vi "Commands.vi"() -> ()   [LabVIEW 2014]
panel:
  in  "Enum":T1(ring)
  in  "Send Command":bool
  out "CheckSum Success":bool
  out "Open Comport Error":bool
  out "ACK Receive Error":bool
  out "Command Sent Error":bool
  out "Response Receive Error":bool
  out "Close Comport Error":bool
  out "ASCII String":string
  out "HEX String":string
  in  "VISA resource name":refnum<visa-resource-name>="COM1"
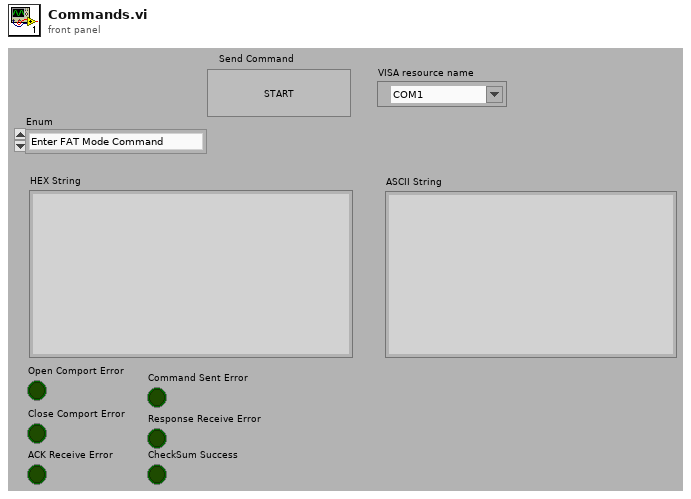
[diagram p1: front panel]
types:
  T1 = enum16{"Enter FAT Mode Command", "Enter Bootstrap Mode Command"}
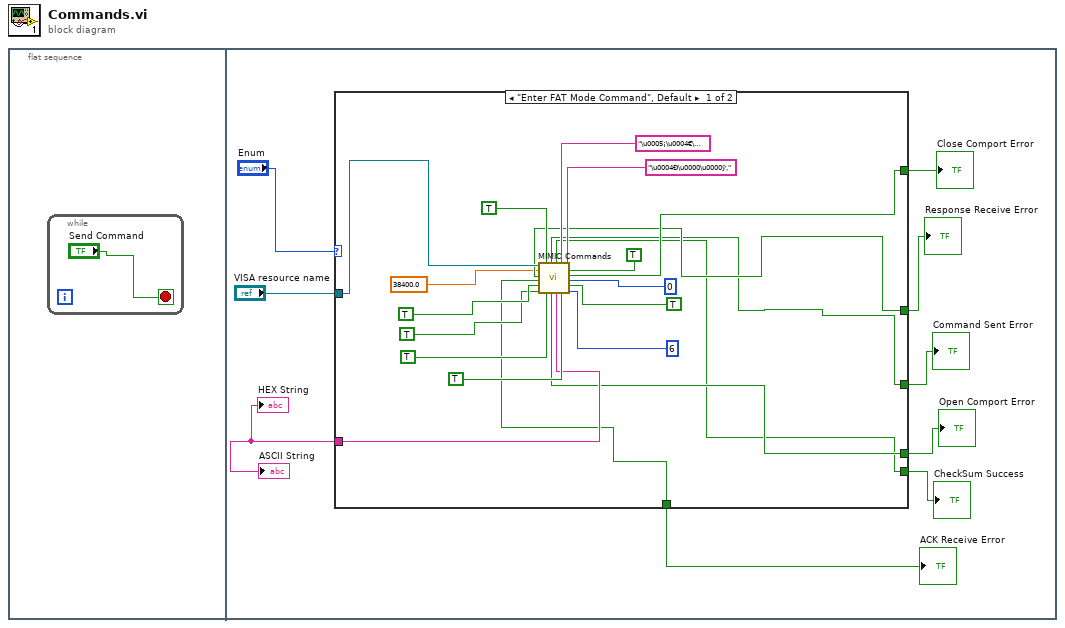
[diagram p0: block diagram]
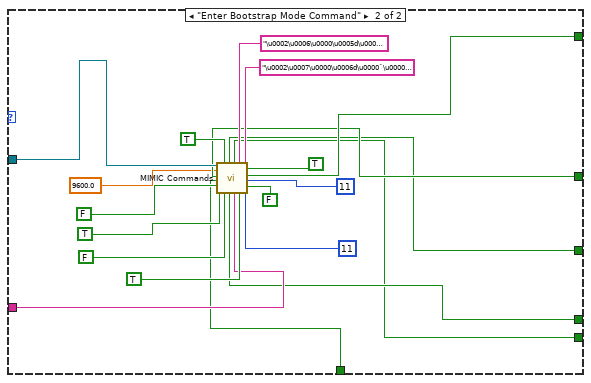
[diagram p2: hidden frame]
diagram:
  n1 = flat-sequence {
    frame #0 {
      n2 = while {
        stop <- "Send Command" stop-if-true
      }
    }
    frame #1 {
      n3 = case shown="\"Enter FAT Mode Command\", Default" "Enum" {
        tunnel: "VISA resource name" -> [w19 w39]
        tunnel: [w18 w38] -> w9
        tunnel: [w17 w37] -> w8
        tunnel: [w16 w36] -> w7
        tunnel: [w15 w35] -> w6
        tunnel: [w14 w34] -> w5
        tunnel: [w13 w33] -> w4
        tunnel: [w12 w32] -> w3
        frame "Enter FAT Mode Command", Default {
          n4 = call "MIMIC Commands.vi"("VISA resource name"=w19, "Baud Rate"=38400.0, "Verify CheckSum"=TRUE, "Read COM Port"=TRUE, "Write to COM Port"=TRUE, "Add CheckSum"=TRUE, "String To Write"="\u0005¡\u0004€\u0010", "Send Command"=TRUE, "ACK HEX String"="\u0004Ð\u0000\u0000ÿ,", "ACK"=TRUE, "Response: bytes to\n read"=u32 0 ("Response: bytes to\n read"), "Response"=TRUE, "ACK: bytes to read"=u32 6) -> ("Response RECEIVE ERROR"=w16:bool, "ACK RECEIVE Error"=w12:bool, "Command SENT Error"=w15:bool, "Open Comport Error"=w14:bool, "CheckSum SUCCESS"=w13:bool, "Response HEX String"=w18:string, "Close Comport Error"=w17:bool)
        }
        frame "Enter Bootstrap Mode Command" {
          n5 = call "MIMIC Commands.vi"("VISA resource name"=w39, "Baud Rate"=9600.0, "Verify CheckSum"=FALSE, "Read COM Port"=TRUE, "Write to COM Port"=TRUE, "Add CheckSum"=FALSE, "String To Write"="\u0002\u0006\u0000\u0005d\u0000\bÿ‰", "Send Command"=TRUE, "ACK HEX String"="\u0002\u0007\u0000\u0006d\u0000ˆ\u0000ÿ\u0007\u0004", "ACK"=TRUE, "Response: bytes to\n read"=u32 11 ("Response: bytes to\n read"), "Response"=FALSE, "ACK: bytes to read"=u32 11) -> ("Response RECEIVE ERROR"=w36:bool, "ACK RECEIVE Error"=w32:bool, "Command SENT Error"=w35:bool, "Open Comport Error"=w34:bool, "CheckSum SUCCESS"=w33:bool, "Response HEX String"=w38:string, "Close Comport Error"=w37:bool)
        }
      }
      "HEX String" <- w9
      "ASCII String" <- w9
      "Close Comport Error" <- w8
      "Response Receive Error" <- w7
      "Command Sent Error" <- w6
      "Open Comport Error" <- w5
      "CheckSum Success" <- w4
      "ACK Receive Error" <- w3
    }
  }
